vi "ESP Set (SubVI).vi"(0 "ESP Config":T1={"COM Port Input"="COM8", "Manual Command"={"Device Type"="", "Instance"="", "Command"="", "Sub-Command"="", "Parameters (Seperate by :)"=""}, "Device Type"="e", "Instance"="a", "Use Manual Command"=TRUE, "Timeout [msec]"=1000, "Read/Write Wait [msec]"=25}, 5 "SET Table Ref":refnum<vi>, 7 "Active SET Commands Ref":refnum<vi>, 14 "Stop Program?":bool) -> (4 "ESP Output":T2={"Write Command"="ea:DU:1", "Read String"="\u0006\u0001ea:00.000:00.000:00.036:00.004:AEA8\u0004", "Read Bytes"=12, "Bytes at Port"=12, "Response"="ea:00.000:00.000:00.036:00.004:AEA8", "ACK"=TRUE, "EOT"=TRUE, "NAK"=FALSE, "Parameters"=["00.000", "00.000", "00.036", "00.004"]}, 15 "ESP Error":errorcluster={"status"=FALSE, "code"=1073676294, "source"="VISA Read in ESP-D Read-Write (SubVI).vi->IO Board Evaluate.vi"})   [LabVIEW 2011]
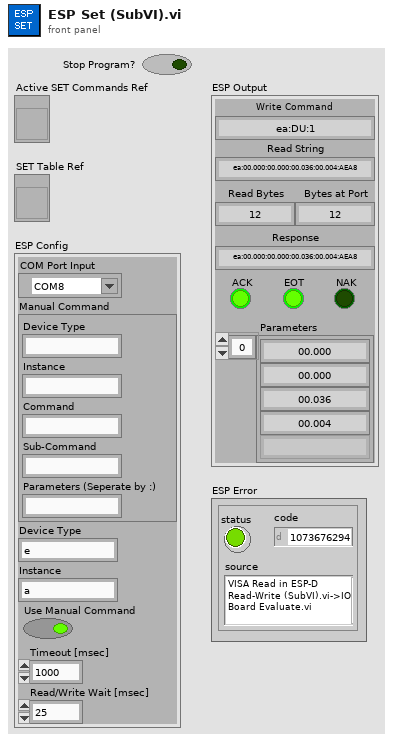
[diagram p1: front panel]
types:
  T1 = cluster{"COM Port Input":refnum<visa-resource-name>, "Manual Command":cluster{"Device Type":string, "Instance":string, "Command":string, "Sub-Command":string, "Parameters (Seperate by :)":string}, "Device Type":string, "Instance":string, "Use Manual Command":bool, "Timeout [msec]":u32, "Read/Write Wait [msec]":u32}
  T2 = cluster{"Write Command":string, "Read String":string, "Read Bytes":u32, "Bytes at Port":u32, "Response":string, "ACK":bool, "EOT":bool, "NAK":bool, "Parameters":string[]}
  T3 = cluster{"Device Type":string, "Instance":string, "Command":string, "Sub-Command":string, "Parameters (Seperate by :)":string}
  T4 = cluster{"CMD_Desc":string, "Param_Names":string[], "Param_Values":string[]}
  T5 = cluster{"CMD_Desc":string, "Param_Names":string[], "Param_Values":string[]}[]
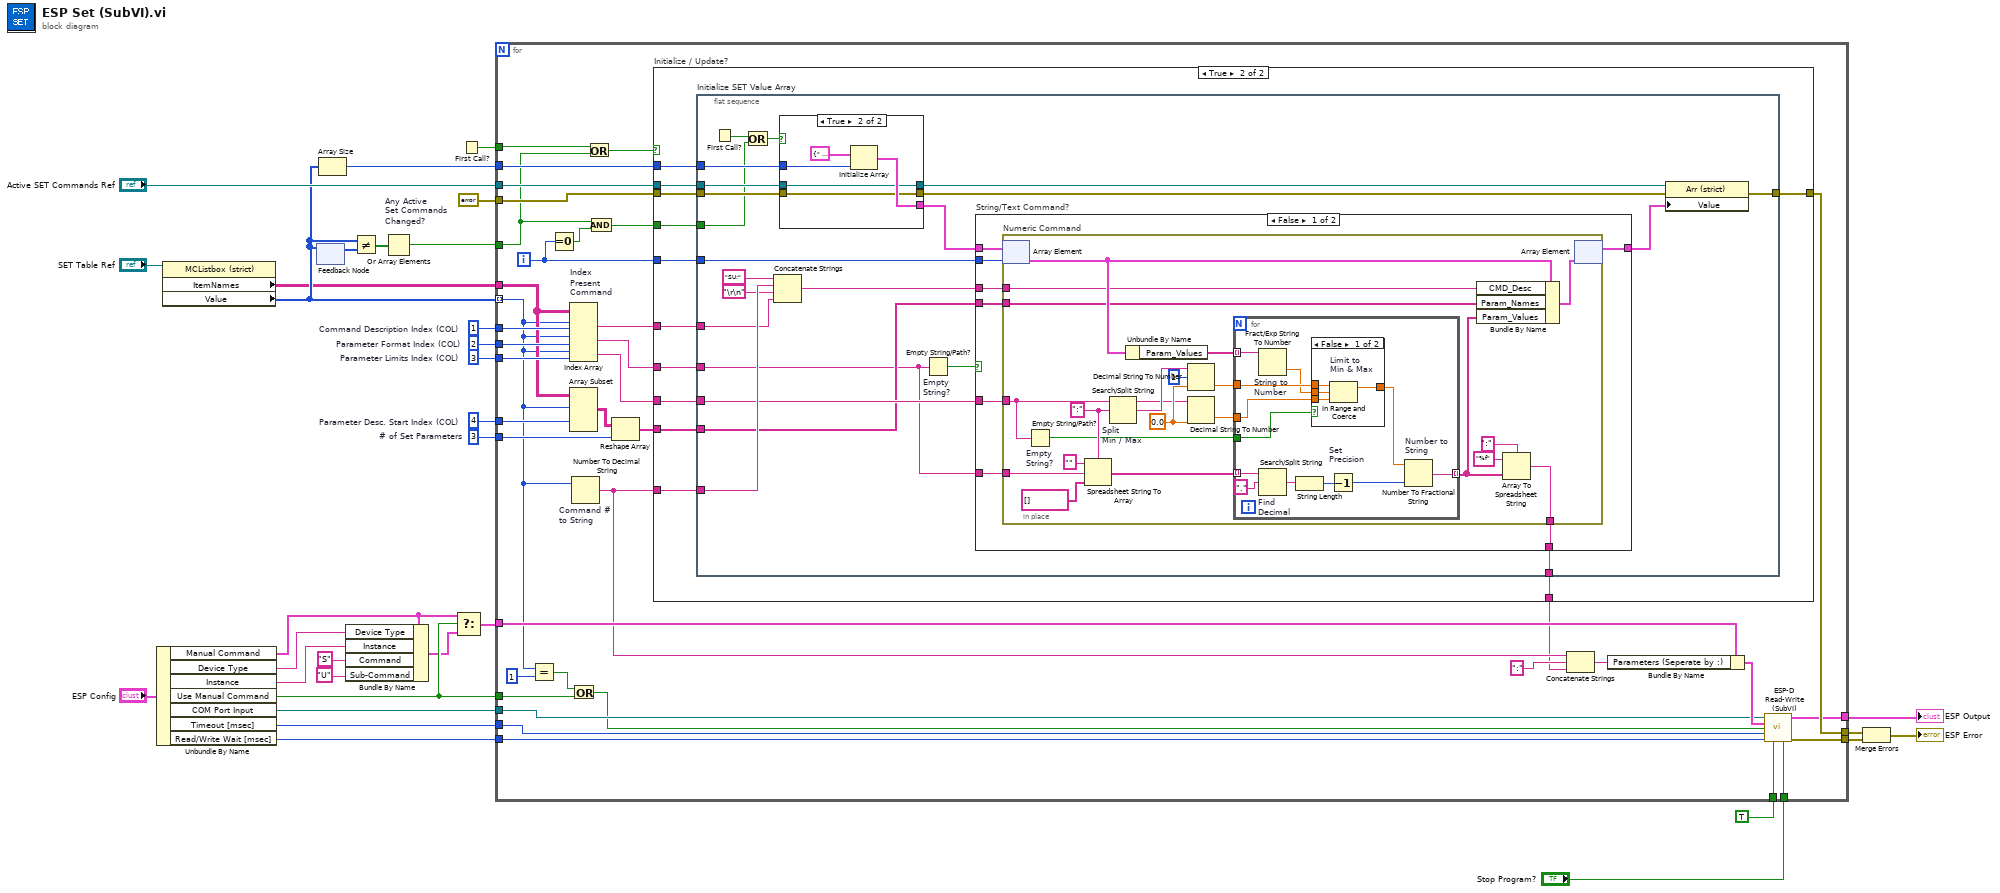
[diagram p0: block diagram]
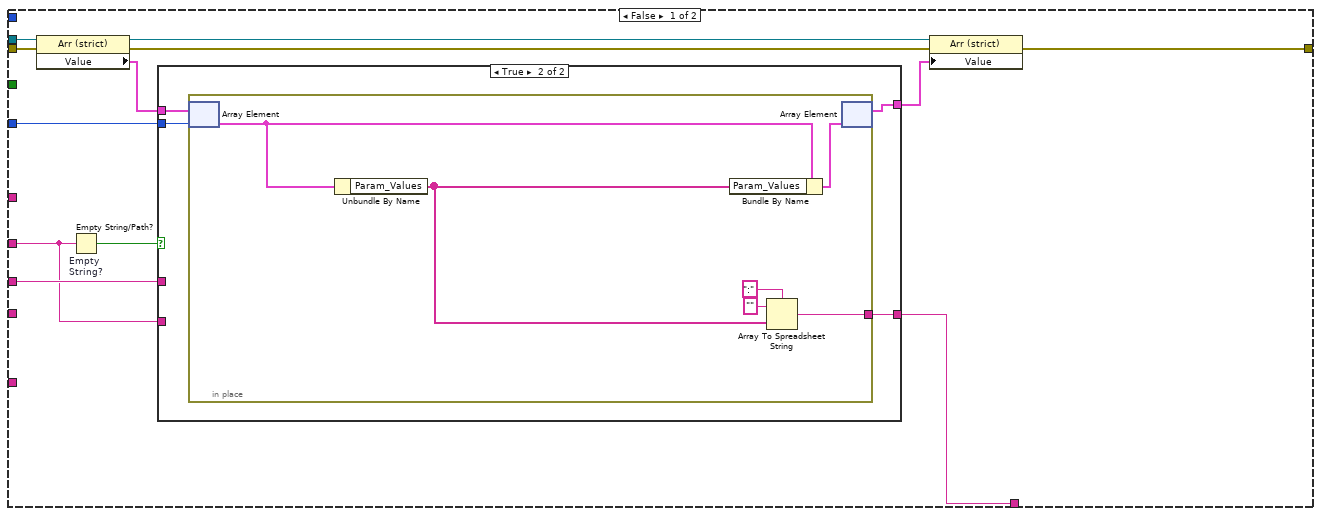
[diagram p2: hidden frame]
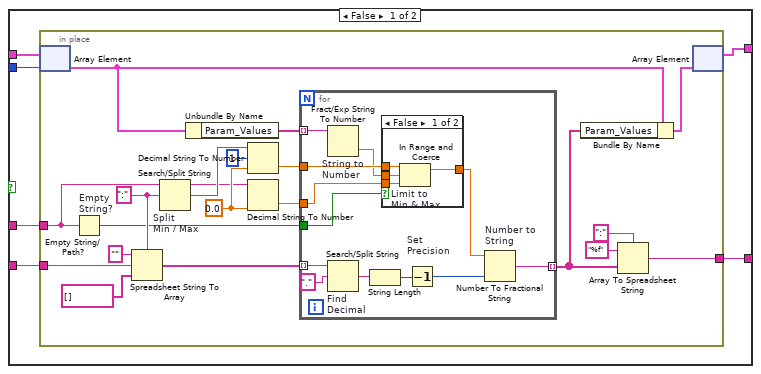
[diagram p3: hidden frame]
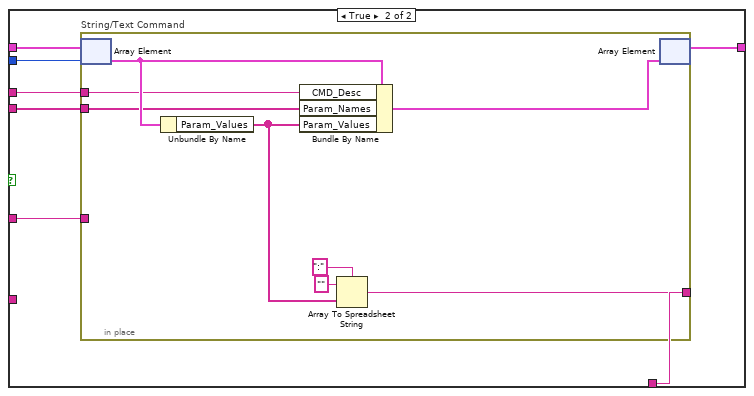
[diagram p6: hidden frame]
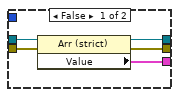
[diagram p7: hidden frame]
diagram:
  w8 = 1  # Command Description Index (COL)
  w5 = 3  # # of Set Parameters
  w6 = 4  # Parameter Desc. Start Index (COL)
  w4 = 3  # Parameter Limits Index (COL)
  w3 = 2  # Parameter Format Index (COL)
  n1 = Unbundle By Name("ESP Config") -> ("Manual Command"=w19:T3, "Device Type"=w21:string, "Instance"=w20:string, "Use Manual Command"=w27:bool, "COM Port Input"=w26:refnum<visa-resource-name>, "Timeout [msec]"=w28:u32, "Read/Write Wait [msec]"=w29:u32)
  n2 = property class="MCListbox (strict)"(reference="SET Table Ref") -> ("ItemNames"=w9:string[][], "Value"=w14:i32[])  [unwired: 1 in, 2 out]
  n3 = feedback #1() -> (w13:i32[])  [unwired: 1 in]
  n4 = feedback-in #1(w14) -> ()
  n5 = Array Size(array=w14) -> (size(s)=w10:i32)
  n6 = Bundle By Name(cluster=w19, "Device Type"=w21, "Instance"=w20, "Command"="S", "Sub-Command"="U") -> (w18:T3)
  n7 = Not Equal?(x=w14, y=w13) -> (x != y?=w12:bool[])
  n8 = Or Array Elements "Any Active\nSet Commands\nChanged?"(Boolean array=w12) -> (logical OR=w15:bool)
  n9 = Select(t=w19, s=w27, f=w18) -> (s? t:f=w24:T3)
  n10 = First Call?() -> (First Call?: T/F=w11:bool)
  n11 = for {
    tunnel: "Active SET Commands Ref" -> [w72]
    tunnel: w3 -> [w70]
    tunnel: w4 -> [w69]
    tunnel: w5 -> [w68]
    tunnel: w6 -> [w67]
    tunnel: errorcluster {"status"=FALSE, "code"=0, "source"=""} ("error in (no error)") -> [w66]
    tunnel: w8 -> [w65]
    tunnel: w14 -> [w42] mode=indexing
    tunnel: w9 -> [w59]
    tunnel: w10 -> [w58]
    tunnel: w11 -> [w53]
    tunnel: w15 -> [w52]
    tunnel: [w51] -> w16
    tunnel: [w50] -> w17
    tunnel: w24 -> [w49]
    tunnel: w26 -> [w46]
    tunnel: w27 -> [w43]
    tunnel: w28 -> [w40]
    tunnel: w29 -> [w39]
    tunnel: [w36] -> w30
    tunnel: "Stop Program?" -> [w35]
    tunnel: TRUE ("Auto-Write on New Command?") -> [w34]
    i -> [w56]
    n12 = Equal?(x=w42, y=1) -> (x = y?=w44:bool)
    n13 = Equal To 0?(x=w56) -> (x = 0?=w57:bool)
    n14 = Index Array "Index\nPresent\nCommand"(array=w59, index (row) #1=w42, index (col) #1=w65, index (row) #2=w42, index (col) #2=w70, index (row) #3=w42, index (col) #3=w69) -> (element #1=w63:string, element #2=w62:string, element #3=w61:string)
    n15 = Array Subset(array=w59, index (row)=w42, index (col)=w67) -> (w71:string[][])  [unwired: 2 in]
    n16 = Or(x=w44, y=w43) -> (x .or. y?=w41:bool)
    n17 = Number To Decimal String "Command #\nto String"(number=w42) -> (decimal integer string=w48:string)  [unwired: 1 in]
    n18 = Or(x=w53, y=w52) -> (x .or. y?=w55:bool)
    n19 = And(x=w52, y=w57) -> (x .and. y?=w54:bool)
    n20 = Reshape Array(w71, w68) -> (w64:string[])
    n21 = case "Initialize / Update?" shown="True" w55 {
      tunnel: w72 -> [w84 w149]
      tunnel: w63 -> [_ w148]
      tunnel: w66 -> [w83 w147]
      tunnel: w56 -> [w75 w145]
      tunnel: [w77 w146] -> w50
      tunnel: w48 -> [_ w144]
      tunnel: w64 -> [_ w143]
      tunnel: w62 -> [w74 w142]
      tunnel: w61 -> [w76 w141]
      tunnel: [w81 w140] -> w37
      tunnel: w58 -> [_ w139]
      tunnel: w54 -> [_ w138]
      frame False {
        n22 = property class="Arr (strict)"(reference=w84, error in=w83) -> (reference out=w80:refnum<vi>, error out=w79:errorcluster, "Value"=w82:T5)
        n23 = Empty String/Path? "Empty\nString?"(string/path=w74) -> (empty?=w73:bool)
        n24 = case shown="True" w73 {
          tunnel: w82 -> [w90 w131]
          tunnel: [w89 w130] -> w81
          tunnel: [w88 w129] -> w78
          tunnel: w74 -> [w87 _]
          tunnel: w76 -> [w86 _]
          tunnel: w75 -> [w85 w128]
          frame False {
            n25 = in-place {
              in-place-border: w87 -> [w99]
              in-place-border: w86 -> [w92]
              in-place-border: [w93] -> w89
              w103 = 0.0
              w110 = ":" ("delimiter (Tab)")
              n26 = in-place-array #2(w90, w85) -> (w96:T4)
              n27 = Empty String/Path? "Empty\nString?"(string/path=w92) -> (empty?=w91:bool)
              n28 = Spreadsheet String To Array(delimiter (Tab)=w110, format string="", spreadsheet string=w99, array type (2D Dbl)=string[] []) -> (array=w108:string[])
              n29 = Search/Split String "Split\nMin / Max"(string=w92, search string/char (-)=w110) -> (substring before match=w102:string, match + rest of string=w104:string)  [unwired: 1 in, 1 out]
              n30 = Unbundle By Name(w96) -> ("Param_Values"=w98:string[])
              n31 = Decimal String To Number(string=w104, offset=1, default (0L)=w103) -> (number=w106:dbl)  [unwired: 1 out]
              n32 = Decimal String To Number(string=w102, default (0L)=w103) -> (number=w107:dbl)  [unwired: 1 in, 1 out]
              n33 = for {
                tunnel: w108 -> [w118] mode=indexing
                tunnel: w106 -> [w120]
                tunnel: w107 -> [w121]
                tunnel: [w114] -> w95 mode=indexing
                tunnel: w98 -> [w112] mode=indexing
                tunnel: w91 -> [w111]
                n34 = Fract/Exp String To Number "String to\nNumber"(string=w112) -> (number=w119:dbl)  [unwired: 3 in, 1 out]
                n35 = Search/Split String "Find\nDecimal"(string=w118, search string/char (-)=".") -> (match + rest of string=w117:string)  [unwired: 1 in, 2 out]
                n36 = String Length(string=w117) -> (length=w115:i32)
                n37 = case shown="False" w111 {
                  tunnel: w121 -> [w126 _]
                  tunnel: w120 -> [w125 _]
                  tunnel: w119 -> [w124 w127]
                  tunnel: [w123 w127] -> w113
                  frame False {
                    n38 = In Range and Coerce "Limit to\nMin & Max"(upper limit=w125, x=w124, lower limit=w126) -> (coerced(x)=w123:dbl)  [unwired: 1 out]
                  }
                  frame True {
                  }
                }
                n39 = Decrement "Set\nPrecision"(x=w115) -> (x-1=w116:i32)
                n40 = Number To Fractional String "Number to\nString"(number=w113, precision (6)=w116) -> (F-format string=w114:string)  [unwired: 2 in]
              }
              n41 = Bundle By Name(cluster=w96, "Param_Values"=w95) -> (w94:T4)
              n42 = Array To Spreadsheet String(delimiter (Tab)=":", array=w95, 3:"%f" ("format string")) -> (spreadsheet string=w93:string)
              n43 = in-place-array #2(w94) -> (w88:T5)  [unwired: 1 out]
            }
          }
          frame True {
            n44 = in-place {
              in-place-border: [w133] -> w130
              n45 = in-place-array #3(w131, w128) -> (w135:T4)
              n46 = Unbundle By Name(w135) -> ("Param_Values"=w132:string[])
              n47 = Bundle By Name(cluster=w135, "Param_Values"=w132) -> (w134:T4)
              n48 = Array To Spreadsheet String(delimiter (Tab)=":", array=w132, 3:"" ("format string")) -> (spreadsheet string=w133:string)
              n49 = in-place-array #3(w134) -> (w129:T5)  [unwired: 1 out]
            }
          }
        }
        n50 = property class="Arr (strict)"(reference=w80, error in=w79, "Value"=w78) -> (error out=w77:errorcluster)  [unwired: 1 out]
      }
      frame True {
        n51 = flat-sequence "Initialize SET Value Array" {
          tunnel: w149 -> [w158]
          tunnel: w148 -> [w168]
          tunnel: w147 -> [w157]
          tunnel: [w171] -> w146
          tunnel: w145 -> [w164]
          tunnel: w144 -> [w170]
          tunnel: w143 -> [w163]
          tunnel: w142 -> [w154]
          tunnel: w141 -> [w166]
          tunnel: [w162] -> w140
          tunnel: w139 -> [w161]
          tunnel: w138 -> [w150]
          frame #0 {
            n52 = First Call?() -> (First Call?: T/F=w151:bool)
            n53 = Or(x=w151, y=w150) -> (x .or. y?=w152:bool)
            n54 = Concatenate Strings("SU:" ("string"), w170, "\r\n", w168) -> (w159:string)
            n55 = case shown="True" w152 {
              tunnel: [w234 w242] -> w165
              tunnel: w161 -> [_ w241]
              tunnel: w158 -> [w238 w240]
              tunnel: w157 -> [w237 w239]
              tunnel: [w236 w240] -> w156
              tunnel: [w235 w239] -> w155
              frame False {
                n56 = property class="Arr (strict)"(reference=w238, error in=w237) -> (reference out=w236:refnum<vi>, error out=w235:errorcluster, "Value"=w234:T5)
              }
              frame True {
                n57 = Initialize Array(T4 {"CMD_Desc"=" ", "Param_Names"=["", "", " "], "Param_Values"=["", "", " "]} ("Cluster 2"), w241) -> (w242:T5)
              }
            }
            n58 = Empty String/Path? "Empty\nString?"(string/path=w154) -> (empty?=w153:bool)
            n59 = case "String/Text Command?" shown="False" w153 {
              tunnel: w154 -> [w179 _]
              tunnel: w166 -> [w178 w225]
              tunnel: w165 -> [w177 w224]
              tunnel: w164 -> [w176 w223]
              tunnel: w163 -> [w175 w222]
              tunnel: [w174 w221] -> w162
              tunnel: [w173 w220] -> w160
              tunnel: w159 -> [w172 w219]
              frame False {
                n60 = in-place "Numeric Command" {
                  in-place-border: w179 -> [w190]
                  in-place-border: w178 -> [w181]
                  in-place-border: w172 -> [w186]
                  in-place-border: w175 -> [w185]
                  in-place-border: [w182] -> w174
                  w194 = 0.0
                  w201 = ":" ("delimiter (Tab)")
                  n61 = in-place-array #4(w177, w176) -> (w187:T4)
                  n62 = Empty String/Path? "Empty\nString?"(string/path=w181) -> (empty?=w180:bool)
                  n63 = Spreadsheet String To Array(delimiter (Tab)=w201, format string="", spreadsheet string=w190, array type (2D Dbl)=string[] []) -> (array=w199:string[])
                  n64 = Search/Split String "Split\nMin / Max"(string=w181, search string/char (-)=w201) -> (substring before match=w193:string, match + rest of string=w195:string)  [unwired: 1 in, 1 out]
                  n65 = Unbundle By Name(w187) -> ("Param_Values"=w189:string[])
                  n66 = Decimal String To Number(string=w195, offset=1, default (0L)=w194) -> (number=w197:dbl)  [unwired: 1 out]
                  n67 = Decimal String To Number(string=w193, default (0L)=w194) -> (number=w198:dbl)  [unwired: 1 in, 1 out]
                  n68 = for {
                    tunnel: w199 -> [w209] mode=indexing
                    tunnel: w197 -> [w211]
                    tunnel: w198 -> [w212]
                    tunnel: [w205] -> w184 mode=indexing
                    tunnel: w189 -> [w203] mode=indexing
                    tunnel: w180 -> [w202]
                    n69 = Fract/Exp String To Number "String to\nNumber"(string=w203) -> (number=w210:dbl)  [unwired: 3 in, 1 out]
                    n70 = Search/Split String "Find\nDecimal"(string=w209, search string/char (-)=".") -> (match + rest of string=w208:string)  [unwired: 1 in, 2 out]
                    n71 = String Length(string=w208) -> (length=w206:i32)
                    n72 = case shown="False" w202 {
                      tunnel: w212 -> [w217 _]
                      tunnel: w211 -> [w216 _]
                      tunnel: w210 -> [w215 w218]
                      tunnel: [w214 w218] -> w204
                      frame False {
                        n73 = In Range and Coerce "Limit to\nMin & Max"(upper limit=w216, x=w215, lower limit=w217) -> (coerced(x)=w214:dbl)  [unwired: 1 out]
                      }
                      frame True {
                      }
                    }
                    n74 = Decrement "Set\nPrecision"(x=w206) -> (x-1=w207:i32)
                    n75 = Number To Fractional String "Number to\nString"(number=w204, precision (6)=w207) -> (F-format string=w205:string)  [unwired: 2 in]
                  }
                  n76 = Bundle By Name(cluster=w187, "CMD_Desc"=w186, "Param_Names"=w185, "Param_Values"=w184) -> (w183:T4)
                  n77 = Array To Spreadsheet String(delimiter (Tab)=":", array=w184, 3:"%f" ("format string")) -> (spreadsheet string=w182:string)
                  n78 = in-place-array #4(w183) -> (w173:T5)  [unwired: 1 out]
                }
              }
              frame True {
                n79 = in-place "String/Text Command" {
                  in-place-border: w225 -> [_]
                  in-place-border: w219 -> [w231]
                  in-place-border: w222 -> [w230]
                  in-place-border: [w228] -> w221
                  n80 = in-place-array #5(w224, w223) -> (w232:T4)
                  n81 = Unbundle By Name(w232) -> ("Param_Values"=w227:string[])
                  n82 = Bundle By Name(cluster=w232, "CMD_Desc"=w231, "Param_Names"=w230, "Param_Values"=w227) -> (w229:T4)
                  n83 = Array To Spreadsheet String(delimiter (Tab)=":", array=w227, 3:"" ("format string")) -> (spreadsheet string=w228:string)
                  n84 = in-place-array #5(w229) -> (w220:T5)  [unwired: 1 out]
                }
              }
            }
            n85 = property class="Arr (strict)"(reference=w156, error in=w155, "Value"=w160) -> (error out=w171:errorcluster)  [unwired: 1 out]
          }
        }
      }
    }
    n86 = Concatenate Strings(w48, ":" ("delimiter (Tab)"), w37) -> (w38:string)
    n87 = Bundle By Name(cluster=w49, "Parameters (Seperate by :)"=w38) -> (w47:T3)
    n88 = call "ESP-D Read-Write (SubVI).vi"("COM Port Input"=w46, "Command Input"=w47, "Manual Write Command"=w41, "Timeout (ms)"=w40, "Write/Read Wait (ms)"=w39, "Auto-Write on New Command?"=w34, "Stop Program?"=w35) -> ("ESP Values"=w36:T2, "Error Output"=w51:errorcluster)  [unwired: 7 in]
  }
  "ESP Output" <- w30
  n89 = Merge Errors(w17, w16) -> (→"ESP Error":errorcluster)
